vi "Integrator 4DOF PID (SubVI).vi"(1 "Reset":bool, 2 "Input":dbl[](array[numeric]), 3 "dt":dbl=0.5) -> (0 "Output":dbl[](array[numeric]))   [LabVIEW 2011]
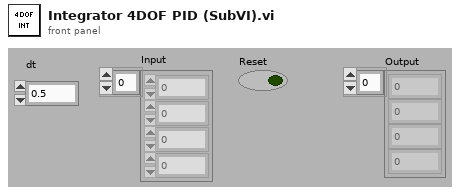
[diagram p1: front panel]
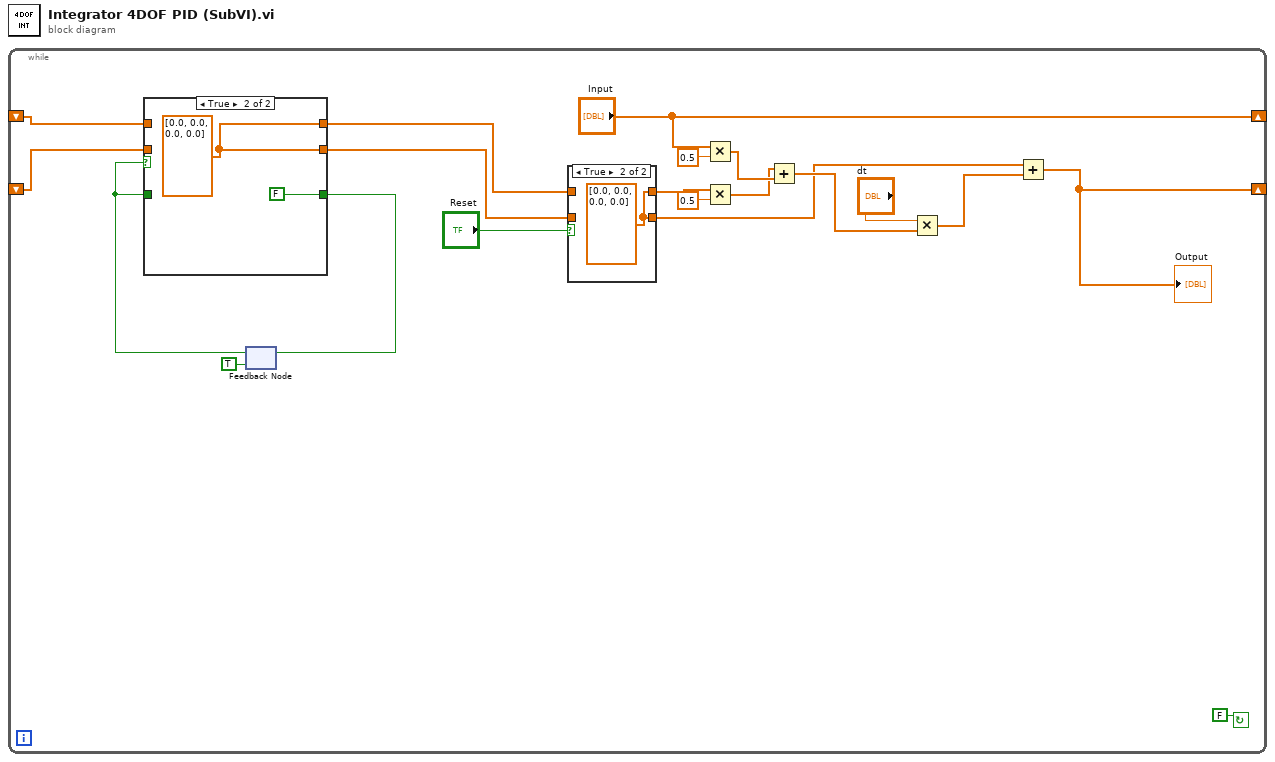
[diagram p0: block diagram]
diagram:
  n1 = while {
    shift-right: [w15] -> _
    shift-left: _ -> [w6]
    shift-right: ["Input"] -> _
    shift-left: _ -> [w7]
    stop <- FALSE continue-if-true
    n2 = feedback #1(TRUE) -> (w2:bool)
    n3 = case shown="True" w2 {
      tunnel: w6 -> [w23 _]
      tunnel: [w23 w25] -> w4
      tunnel: w7 -> [w22 _]
      tunnel: [w22 w25] -> w5
      tunnel: [w21 FALSE] -> w3
      tunnel: w2 -> [w21 _]
      frame False {
      }
      frame True {
        w25 = dbl[] [0.0, 0.0, 0.0, 0.0] ("Input")
      }
    }
    n4 = feedback-in #1(w3) -> ()
    n5 = case shown="True" "Reset" {
      tunnel: w4 -> [w27 _]
      tunnel: [w27 w28] -> w13
      tunnel: w5 -> [w26 _]
      tunnel: [w26 w28] -> w8
      frame False {
      }
      frame True {
        w28 = dbl[] [0.0, 0.0, 0.0, 0.0] ("Input")
      }
    }
    n6 = Multiply(x="Input", y=0.5) -> (x*y=w19:dbl[])
    n7 = Multiply(x=w8, y=0.5) -> (x*y=w17:dbl[])
    n8 = Add(x=w17, y=w19) -> (x+y=w16:dbl[])
    n9 = Multiply(x="dt", y=w16) -> (x*y=w11:dbl[])
    n10 = Add(x=w13, y=w11) -> (x+y=w15:dbl[])
    "Output" <- w15
  }
